vi "Set Scalar Channel Data.vi"(8 "error in (no error)":errorcluster, 9 "scalar channel in":T1 {"Data Type" format="%.0x"}, 11 "item ref in":T3 format="%.0x") -> (0 "error out":errorcluster, 1 "scalar channel data out":T4 {"Item Ref" format="%.0x"}, 2 "scalar channel out":T1 {"Data Type" format="%.0x"}, 3 "item ref out":T3 format="%.0x")   [LabVIEW 2018, in "FPGA Addon System Explorer.lvlib"]
uses:
  FPGA Addon System Explorer.lvlib
  <vilib>/NI Veristand/Custom Device API/Custom Device Item Ref.ctl
  Addon Shared/Types/Register Information.ctl
  Addon Shared/Types/Data Type.ctl
  Types/Output Scalar.ctl
  <vilib>/NI Veristand/Custom Device API/Custom Device API.lvlib
  Addon Shared/FPGA Addon Shared.lvlib
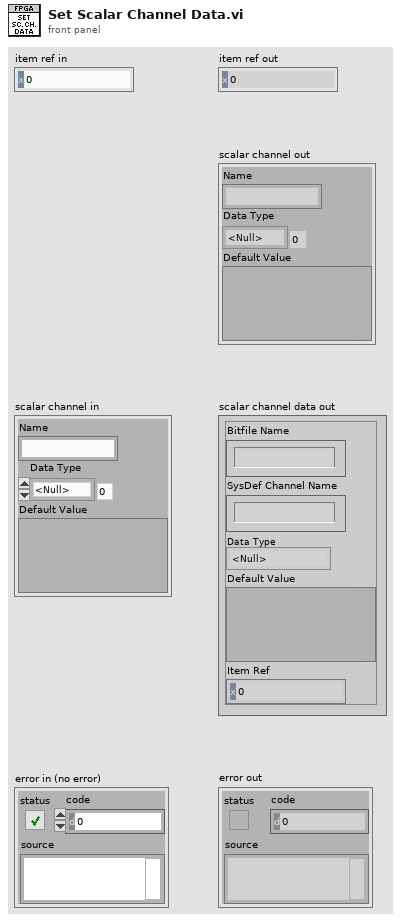
[diagram p1: front panel]
types:
  T1 = typedef "FPGA Addon Shared.lvlib/Register Information.ctl" = cluster{"Name":string, "Data Type":T2, "Default Value":variant}
  T2 = typedef "FPGA Addon Shared.lvlib/Data Type.ctl" = enum8{"<Null>", "I8", "I16", "I32", "I64", "U8", "U16", "U32", "U64", "SGL", "Boolean", "Analog PWM In Settings", "Analog PWM In", "Digital PWM In Settings", "Digital PWM In", "Digital PWM Out", "Sine Out", "FXP+/-24.5", "FXP+/-16.5", "FXP+/-32.8", "FXP+/-64.32", "FXP+/-16.7", "FXP+/-20.5", "FXP+/-27.5", "FXP+/-32.16", "FXP+16.3", "FXP+18.3", "Digital Static In", "Digital Static Out", "Digital Static In Settings", "Digital WSS Out", "Quad Encoder Settings", "Quad Encoder In", "Group"}
  T3 = typedef "Custom Device API.lvlib/Custom Device Item Ref.ctl" = u64
  T4 = typedef "FPGA Addon System Explorer.lvlib/Output Scalar.ctl" = cluster{"Bitfile Name":string, "SysDef Channel Name":string, "Data Type":T2, "Default Value":variant, "Item Ref":T3}
  T5 = typedef "Custom Device API.lvlib/Custom Device Item Info.ctl" = cluster{"Name":string, "Is Channel":bool, "GUID":string, "Is Waveform":bool}
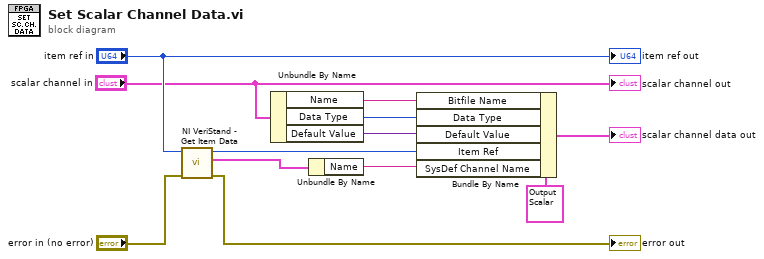
[diagram p0: block diagram]
diagram:
  n1 = call <vilib>:"NI VeriStand - Get Item Data.vi"("error in (no error)"="error in (no error)", "Item Ref in"="item ref in") -> ("error out"=→"error out":errorcluster, "Item Info"=w9:T5, "Item Ref out"=w7:T3)  [unwired: 6 in, 1 out]
  n2 = Unbundle By Name("scalar channel in") -> ("Name"=w1:string, "Data Type"=w2:T2, "Default Value"=w3:variant)
  n3 = Unbundle By Name(w9) -> ("Name"=w8:string)
  n4 = Bundle By Name(cluster=T4 {"Bitfile Name"="", "SysDef Channel Name"="", "Data Type"=enum."<Null>", "Default Value"=variant, "Item Ref"=0} ("Output Scalar data"), "Bitfile Name"=w1, "Data Type"=w2, "Default Value"=w3, "Item Ref"=w7, "SysDef Channel Name"=w8) -> (→"scalar channel data out":T4)
  "item ref out" <- "item ref in"
  "scalar channel out" <- "scalar channel in"
